vi "position to velocity.vi"(6 "first block?":bool, 8 "sampling rate":dbl, 9 "pulse per revolution":i32=2000, 10 "last position":dbl, 11 "position":dbl[](array[numeric]) format="%0.2f") -> (2 "last position out":dbl, 3 "velocity (rpm)":dbl[](array[numeric]) format="%0.2f")   [LabVIEW 2021]
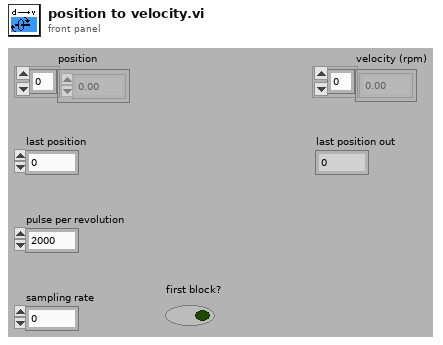
[diagram p1: front panel]
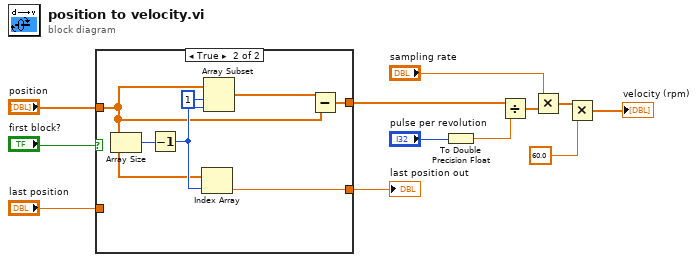
[diagram p0: block diagram]
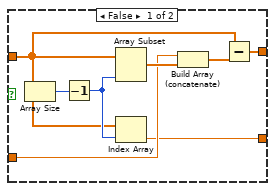
[diagram p2: hidden frame]
diagram:
  n1 = case shown="True" "first block?" {
    tunnel: "last position" -> [w15 _]
    tunnel: "position" -> [w16 w22]
    tunnel: [w14 w27] -> w10
    tunnel: [w13 w26] -> w8
    frame False {
      n2 = Array Size(array=w16) -> (size(s)=w20:i32)
      n3 = Decrement(x=w20) -> (x-1=w17:i32)
      n4 = Array Subset(array=w16, length=w17) -> (w19:dbl[])  [unwired: 1 in]
      n5 = Index Array(array=w16, index=w17) -> (element=w14:dbl)
      n6 = Build Array (concatenate)(w15, w19) -> (w18:dbl[])
      n7 = Subtract(x=w16, y=w18) -> (x-y=w13:dbl[])
    }
    frame True {
      n8 = Array Size(array=w22) -> (size(s)=w25:i32)
      n9 = Decrement(x=w25) -> (x-1=w24:i32)
      n10 = Index Array(array=w22, index=w24) -> (element=w27:dbl)
      n11 = Array Subset(array=w22, index=1, length=w24) -> (w21:dbl[])
      n12 = Subtract(x=w21, y=w22) -> (x-y=w26:dbl[])
    }
  }
  "last position out" <- w10
  n13 = To Double Precision Float(number="pulse per revolution") -> (double precision float=w7:dbl)
  n14 = Divide(x=w8, y=w7) -> (x/y=w6:dbl[])
  n15 = Multiply(x="sampling rate", y=w6) -> (x*y=w4:dbl[])
  n16 = Multiply(x=w4, y=60.0) -> (x*y=→"velocity (rpm)":dbl[])
